vi "Valid.vi"(8 "error in (no error)":errorcluster, 11 "Shared Options in":refnum<class "Shared Options.lvclass">) -> (0 "error out":errorcluster, 2 "Valid":bool, 3 "Shared Options out":refnum<class "Shared Options.lvclass">)   [LabVIEW 2020, in "AutoComplete.lvlib" / "Shared Options.lvclass"]
doc: "Determines if the Shared Options is a valid initialized instance. Used internally to decide between using local handling or shared options configuration."
uses:
  Shared Options.lvclass
  Shared Options.lvclass/Shared Options.ctl
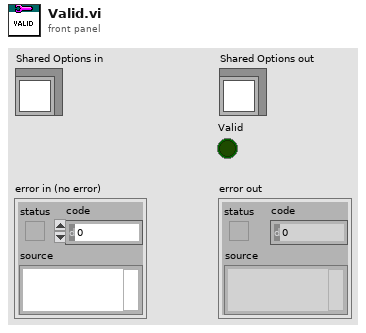
[diagram p1: front panel]
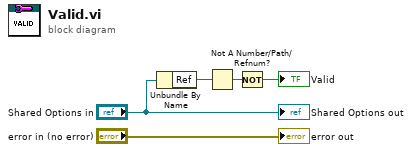
[diagram p0: block diagram]
diagram:
  n1 = Unbundle By Name("Shared Options in") -> ("Ref"=w3:refnum<data-value>)
  n2 = Not A Number/Path/Refnum?(number/path/refnum=w3) -> (NaN/Path/Refnum?=w2:bool)
  n3 = Not(x=w2) -> (.not. x?=→"Valid":bool)
  "error out" <- "error in (no error)"
  "Shared Options out" <- "Shared Options in"
